vi "b-field result sensor0.vi"(9 "position?":bool, 10 "mag0 data":T2[](array[typedef]), 11 "orbit parameters":T4) -> (2 "sensor0 predicted field":dbl[][](array[numeric]), 3 "sensor0 field as reading array":T2[](array[typedef]))   [LabVIEW 2017]
uses:
  typedefs/orbit parameters with crossing info.ctl
  typedefs/reading.ctl
  typedefs/readingType.ctl
  typedefs/orbit magnetic field data.ctl
  typedefs/magnetomter reading set.ctl
panel:
  out "Waveform Graph":dbl[][](graph)
  out "XY Graph":T1(graph)
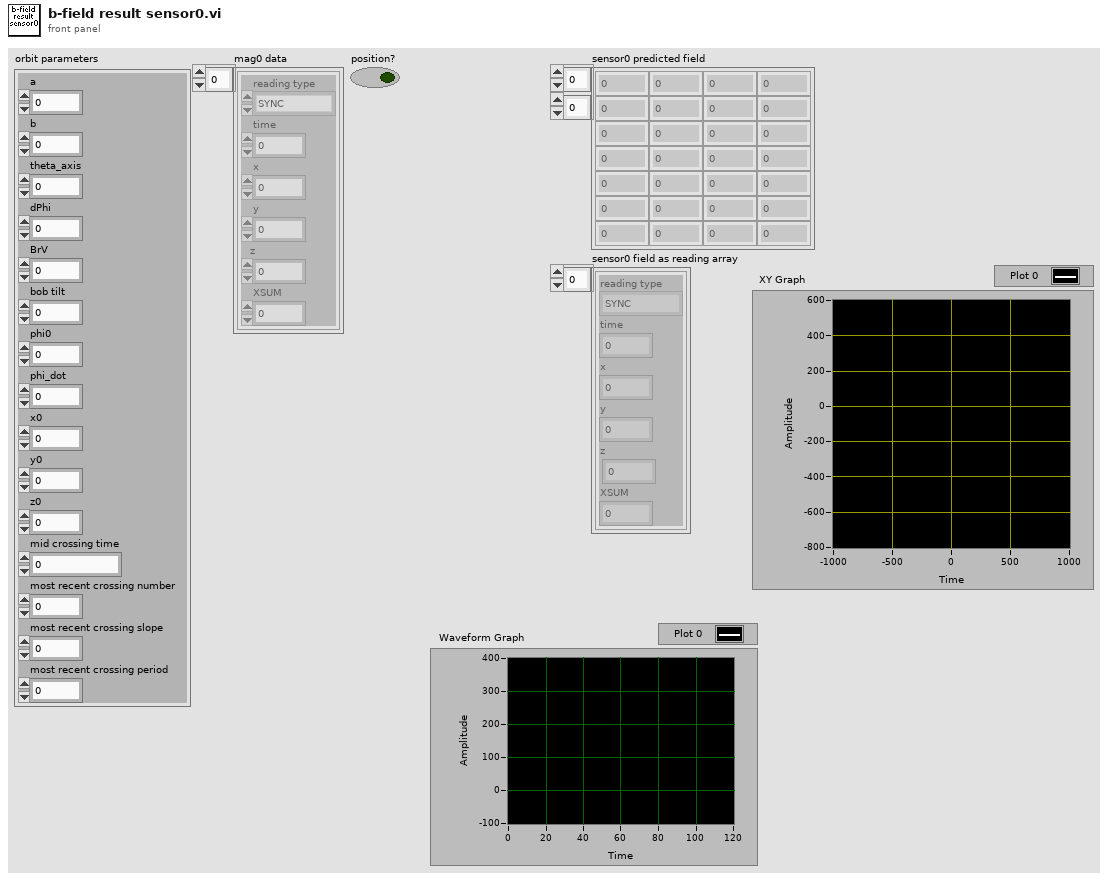
[diagram p1: front panel]
types:
  T1 = cluster{"sensor0 prediction":dbl[], "sensor0 prediction":dbl[]}[]
  T2 = typedef "reading.ctl" = cluster{"reading type":T3, "time":fxp<+,48,48>, "x":sgl, "y":sgl, "z":sgl, "XSUM":u8}
  T3 = typedef "readingType.ctl" = enum8{"SYNC", "DETVAL", "COILI", "MAGVEC", "ACCVEC", "CROSSING", "MAGVEC0", "MAGVEC1", "MAGVEC2", "MAGVEC3", "MAGVEC4", "MAGVEC5", "MAGVEC6", "MAGVEC7"}
  T4 = typedef "orbit parameters with crossing info.ctl" = cluster{"a":dbl, "b":dbl, "theta_axis":dbl, "dPhi":dbl, "BrV":dbl, "bob tilt":dbl, "phi0":dbl, "phi_dot":dbl, "x0":dbl, "y0":dbl, "z0":dbl, "mid crossing time":dbl, "most recent crossing number":dbl, "most recent crossing slope":dbl, "most recent crossing period":dbl}
  T5 = typedef "orbit magnetic field data.ctl" = cluster{"magnetometer readings":T6[], "L":dbl, "omega":dbl, "t0":dbl}
  T6 = typedef "magnetomter reading set.ctl" = cluster{"time":fxp<+,48,48>, "mag readings":cluster{"magnetometer index":dbl, "Bx":dbl, "By":dbl, "Bz":dbl, "magnetometer x":dbl, "magnetometer y":dbl}[]}
  T7 = cluster{"magnetometer index":dbl, "Bx":dbl, "By":dbl, "Bz":dbl, "magnetometer x":dbl, "magnetometer y":dbl}
  T8 = cluster{"magnetometer index":dbl, "Bx":dbl, "By":dbl, "Bz":dbl, "magnetometer x":dbl, "magnetometer y":dbl}[]
  T9 = cluster{"orbit parameters[0]":dbl, "orbit parameters[1]":dbl, "orbit parameters[2]":dbl, "orbit parameters[3]":dbl, "orbit parameters[4]":dbl, "orbit parameters[5]":dbl, "orbit parameters[6]":dbl, "orbit parameters[7]":dbl, "orbit parameters[8]":dbl, "orbit parameters[9]":dbl, "orbit parameters[10]":dbl}
  T10 = cluster{"sensor0 measured":dbl[], "sensor0 measured":dbl[]}
  T11 = cluster{"sensor0 prediction":dbl[], "sensor0 prediction":dbl[]}
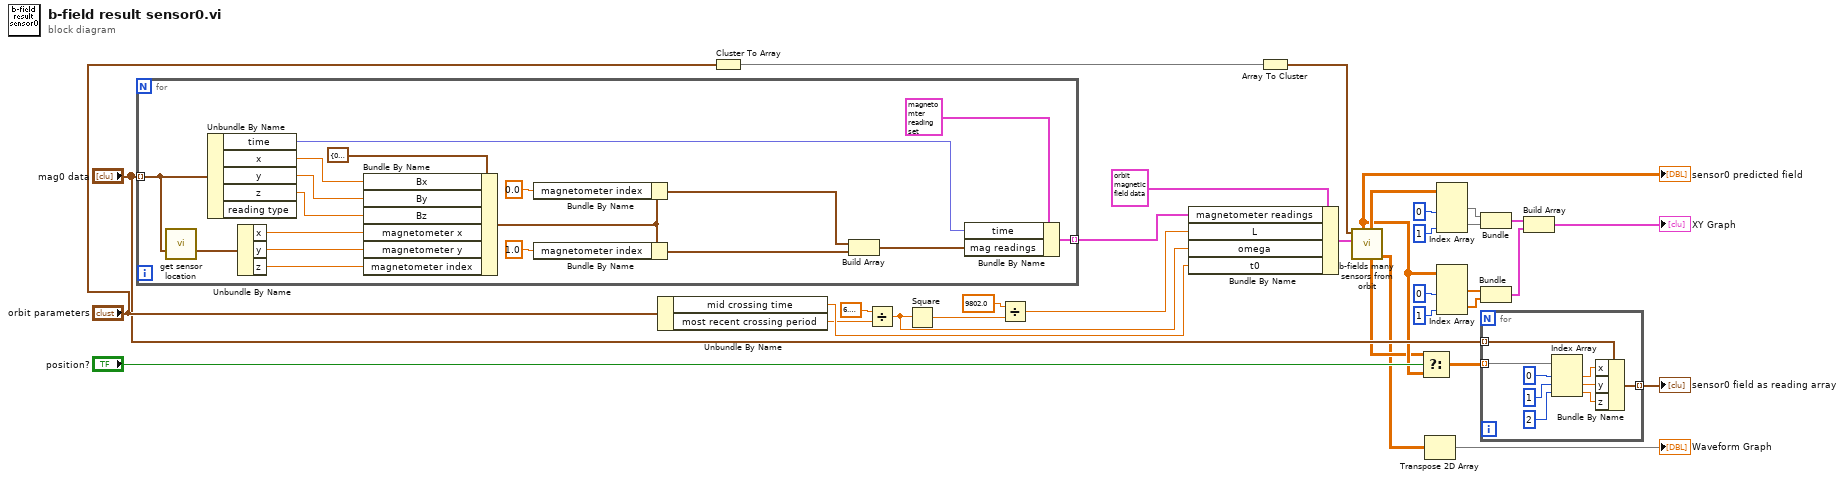
[diagram p0: block diagram]
diagram:
  n1 = for {
    tunnel: "mag0 data" -> [w41] mode=indexing
    tunnel: [w44] -> w30 mode=indexing
    n2 = call "get sensor location.vi"("reading"=w41) -> ("location"=w40:cluster{"x":dbl, "y":dbl, "z":dbl})  [unwired: 14 in]
    n3 = Unbundle By Name(w41) -> ("time"=w49:fxp<+,48,48>, "x"=w48:sgl, "y"=w47:sgl, "z"=w46:sgl)  [unwired: 1 out]
    n4 = Unbundle By Name(w40) -> ("x"=w39:dbl, "y"=w38:dbl, "z"=w37:dbl)
    n5 = Bundle By Name(cluster=T7 {"magnetometer index"=0.0, "Bx"=0.0, "By"=0.0, "Bz"=0.0, "magnetometer x"=0.0, "magnetometer y"=0.0} ("mag readings"), "Bx"=w48, "By"=w47, "Bz"=w46, "magnetometer x"=w39, "magnetometer y"=w38, "magnetometer index"=w37) -> (w36:T7)
    n6 = Bundle By Name(cluster=w36, "magnetometer index"=0.0) -> (w35:T7)
    n7 = Bundle By Name(cluster=w36, "magnetometer index"=1.0) -> (w42:T7)
    n8 = Build Array(w35, w42) -> (w45:T8)
    n9 = Bundle By Name(cluster=T6 {"time"=93283733019.0, "mag readings"=[{"magnetometer index"=0.0, "Bx"=-438.3019714355469, "By"=-49.17140197753906, "Bz"=-1269.87353515625, "magnetometer x"=0.0, "magnetometer y"=0.0}, {"magnetometer index"=1.0, "Bx"=-241.18035888671875, "By"=270.41705322265625, "Bz"=-130.9935302734375, "magnetometer x"=-22.5, "magnetometer y"=38.971}, {"magnetometer index"=2.0, "Bx"=-208.7041015625, "By"=-255.4169921875, "Bz"=-108.7998046875, "magnetometer x"=-22.5, "magnetometer y"=-38.971}, {"magnetometer index"=3.0, "Bx"=562.134765625, "By"=-12.9853515625, "Bz"=-439.384765625, "magnetometer x"=45.0, "magnetometer y"=0.0}]} ("Magnetometer reading set"), "time"=w49, "mag readings"=w45) -> (w44:T6)
  }
  n10 = Unbundle By Name("orbit parameters") -> ("mid crossing time"=w28:dbl, "most recent crossing period"=w26:dbl)
  n11 = Cluster To Array(cluster="orbit parameters") -> (array=w33:dbl[])
  n12 = Divide(x=6.283185307179586, y=w26) -> (x/y=w25:dbl)
  n13 = Square(x=w25) -> (x^2=w24:dbl)
  n14 = Divide(x=9802.0, y=w24) -> (x/y=w22:dbl)
  n15 = Bundle By Name(cluster=T5 data[23284B] ("orbit magnetic field data"), "magnetometer readings"=w30, "L"=w22, "omega"=w25, "t0"=w28) -> (w21:T5)
  n16 = Array To Cluster(array=w33) -> (cluster=w32:T9)
  n17 = call "b-fields many sensors from orbit.vi"("orbit magnetic field data"=w21, "orbit parameters"=w32) -> ("position"=w1:dbl[][], "predicted location"=w3:dbl[][], "sensor0 measured"=w5:dbl[][], "sensor0 prediction"=w4:dbl[][])  [unwired: 3 in, 3 out]
  "sensor0 predicted field" <- w4
  n18 = Select(t=w3, s="position?", f=w4) -> (s? t:f=w18:dbl[][])
  n19 = Transpose 2D Array(2D array=w1) -> (transposed array=→"Waveform Graph":dbl[][])
  n20 = Index Array(array=w5, index (col) #1=0 ("disabled index (col)"), index (col) #2=1 ("index (col)")) -> (element #1=w10:dbl[], element #2=w9:dbl[])  [unwired: 2 in]
  n21 = Index Array(array=w4, index (col) #1=0 ("disabled index (col)"), index (col) #2=1 ("index (col)")) -> (element #1=w14:dbl[], element #2=w13:dbl[])  [unwired: 2 in]
  n22 = Bundle("sensor0 measured"=w10, "sensor0 measured"=w9) -> (w8:T10)  [unwired: 1 in]
  n23 = Bundle("sensor0 prediction"=w14, "sensor0 prediction"=w13) -> (w7:T11)  [unwired: 1 in]
  n24 = for {
    tunnel: "mag0 data" -> [w60] mode=indexing
    tunnel: w18 -> [w59] mode=indexing
    tunnel: [w52] -> w19 mode=indexing
    n25 = Index Array(array=w59, index #1=0 ("index"), index #2=1 ("index"), index #3=2 ("index")) -> (element #1=w55:dbl, element #2=w54:dbl, element #3=w53:dbl)
    n26 = Bundle By Name(cluster=w60, "x"=w55, "y"=w54, "z"=w53) -> (w52:T2)
  }
  "sensor0 field as reading array" <- w19
  n27 = Build Array(w8, w7) -> (→"XY Graph":T1)
